vi "Get Var.vi"(8 "error in (no error)":errorcluster caption="错误输入（无错误）", 11 "Contstant Base输入":refnum<class "Tag Data.lvclass">) -> (0 "error out":errorcluster caption="错误输出", 2 "Var":variant, 3 "Contstant Base输出":refnum<class "Tag Data.lvclass">)   [LabVIEW 2013, in "Tag Data.lvclass"]
uses:
  Tag Data.lvclass
  Tag Data.lvclass/Tag Data.ctl
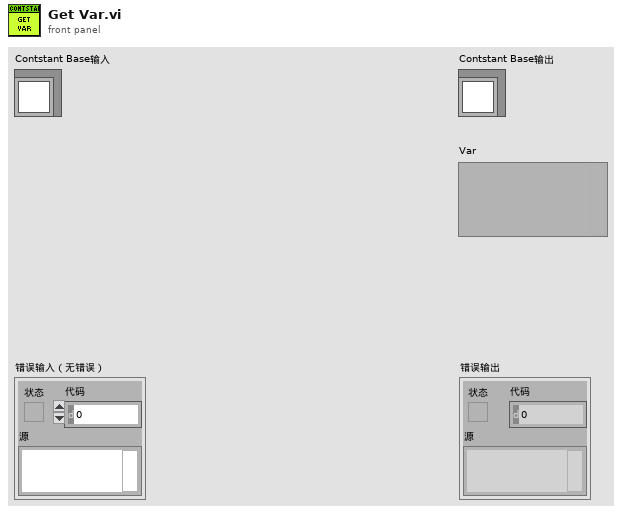
[diagram p1: front panel]
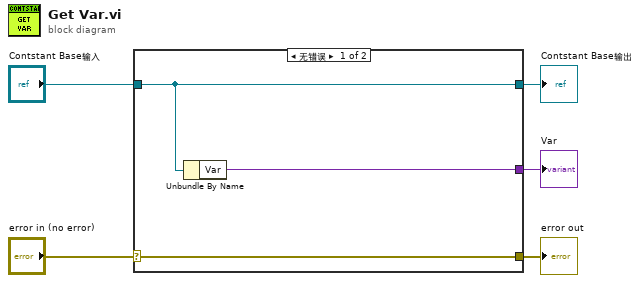
[diagram p0: block diagram]
diagram:
  n1 = case shown="无错误" "error in (no error)" {
    selector: "error in (no error)" -> [w8 w9]
    tunnel: [w8 w9] -> w4
    tunnel: [w7 w10] -> w2
    tunnel: "Contstant Base输入" -> [w7 w10]
    tunnel: [w6 _] -> w1
    frame No Error {
      n2 = Unbundle By Name(w7) -> ("Var"=w6:variant)
    }
    frame Error {
    }
  }
  "error out" <- w4
  "Contstant Base输出" <- w2
  "Var" <- w1
